vi "Rohde & Schwarz VNA Read Trace Display.vi"(4 "Trace":i8=1 min=1 max=99 step=1, 6 "Channel":i8=1 min=1 max=99 step=1, 7 "Rohde & Schwarz VNA":T1, 8 "error in (no error)":errorcluster, 11 "VISA Resource Name":refnum<visa-resource-name>) -> (0 "error out":errorcluster, 1 "Trace Index":i32, 2 "Displayed?":bool, 3 "dup VISA Resource Name":refnum<visa-resource-name>)   [LabVIEW 2011]
uses:
  TypeDefs/Rohde & Schwarz VNA Instrument Info.ctl
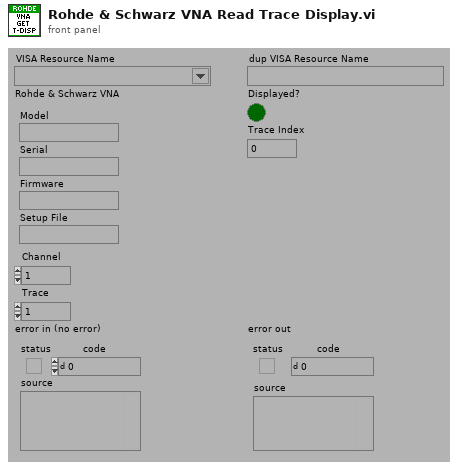
[diagram p1: front panel]
types:
  T1 = typedef "Rohde & Schwarz VNA Instrument Info.ctl" = cluster{"Model":string, "Serial":string, "Firmware":string, "Setup File":string}
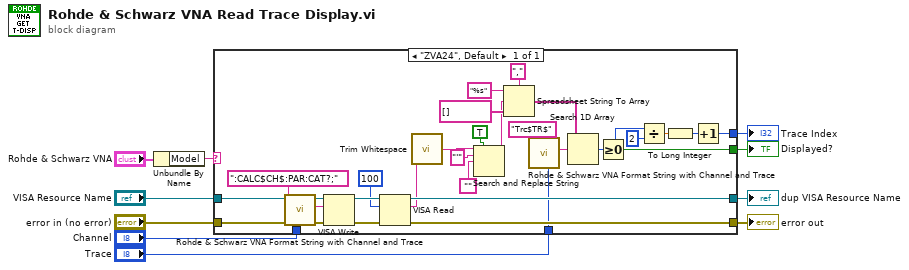
[diagram p0: block diagram]
diagram:
  n1 = Unbundle By Name("Rohde & Schwarz VNA") -> ("Model"=w2:string)
  n2 = case shown="\"ZVA24\", Default" w2 {
    tunnel: "VISA Resource Name" -> [w39]
    tunnel: "error in (no error)" -> [w38]
    tunnel: [w35] -> w8
    tunnel: [w34] -> w7
    tunnel: [w16] -> w6
    tunnel: "Channel" -> [w30]
    tunnel: "Trace" -> [w19]
    tunnel: [w12] -> w1
    frame "ZVA24", Default {
      n3 = call "Rohde & Schwarz VNA Format String with Channel and Trace.vi"("Channel"=w30, "String"=":CALC$CH$:PAR:CAT?;" ("write buffer")) -> ("String Out"=w31:string)  [unwired: 1 in, 6 out]
      n4 = VISA Write(VISA resource name=w39, write buffer=w31, error in (no error)=w38) -> (VISA resource name out=w36:refnum<visa-resource-name>, error out=w37:errorcluster)  [unwired: 1 out]
      n5 = VISA Read(VISA resource name=w36, byte count=u32 100, error in (no error)=w37) -> (VISA resource name out=w35:refnum<visa-resource-name>, read buffer=w21:string, error out=w34:errorcluster)  [unwired: 1 out]
      n6 = call <vilib>:"Trim Whitespace.vi"("string"=w21) -> ("trimmed string"=w22:string)  [unwired: 1 in]
      n7 = Search and Replace String(replace all?=TRUE ("replace all? (F)"), input string=w22, search string="'", replace string="") -> (result string=w23:string)  [unwired: 1 in, 6 out]
      n8 = Spreadsheet String To Array(delimiter (Tab)=",", format string="%s", spreadsheet string=w23, array type (2D Dbl)=string[] []) -> (array=w20:string[])
      n9 = call "Rohde & Schwarz VNA Format String with Channel and Trace.vi"("Trace"=w19, "String"="Trc$TR$" ("format string")) -> ("String Out"=w17:string)  [unwired: 1 in, 6 out]
      n10 = Search 1D Array(1D array=w20, element=w17) -> (index of element=w15:i32)  [unwired: 1 out]
      n11 = Greater Or Equal To 0?(x=w15) -> (x >= 0?=w16:bool)
      n12 = Divide(x=w15, y=2) -> (x/y=w14:dbl)
      n13 = To Long Integer(number=w14) -> (32bit integer=w13:i32)
      n14 = Increment(x=w13) -> (x+1=w12:i32)
    }
  }
  "dup VISA Resource Name" <- w8
  "error out" <- w7
  "Displayed?" <- w6
  "Trace Index" <- w1
